vi "bypass control.vi"(8 "Joystick":dbl, 11 "MotorInput":dbl) -> (3 "SetMotor":dbl)   [LabVIEW 2013]
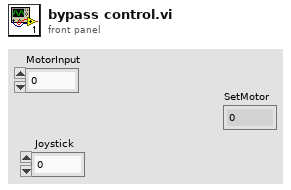
[diagram p1: front panel]
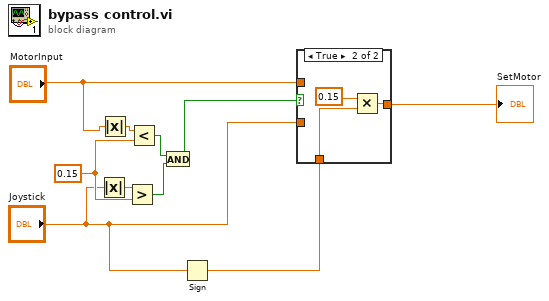
[diagram p0: block diagram]
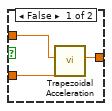
[diagram p2: hidden frame]
diagram:
  w10 = 0.15
  n1 = Absolute Value(x="Joystick") -> (abs(x)=w8:dbl)
  n2 = Absolute Value(x="MotorInput") -> (abs(x)=w9:dbl)
  n3 = Greater?(x=w8, y=w10) -> (0:w6:bool)
  n4 = Less?(x=w9, y=w10) -> (x < y?=w7:bool)
  n5 = And(x=w7, y=w6) -> (x .and. y?=w5:bool)
  n6 = Sign(1:"Joystick") -> (0:w3:dbl)
  n7 = case shown="True" w5 {
    tunnel: "Joystick" -> [w12 _]
    tunnel: "MotorInput" -> [w13 _]
    tunnel: [w11 w16] -> w2
    tunnel: w3 -> [_ w14]
    frame False {
      n8 = call "Trapezoidal Acceleration.vi"("Desired"=w12, "Actual"=w13) -> ("New Actual"=w11:dbl)  [unwired: 9 in]
    }
    frame True {
      n9 = Multiply(x=0.15, y=w14) -> (x*y=w16:dbl)
    }
  }
  "SetMotor" <- w2
